vi "5-CopyFileContent.vi"() -> ()   [LabVIEW 2016, in "TestVIs.lvlib"]
uses:
  TestVIs.lvlib
panel:
  in  "Empty File":path=path "D:/Git/CSPP_MessageMaker/_CSPP_MessageMaker/TestVIs/TestTarget.vi"
  in  "File to Copy":path
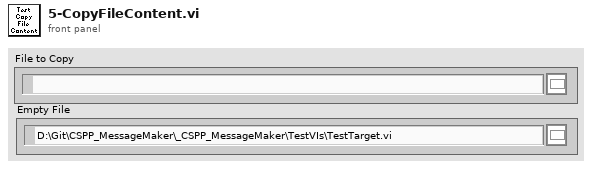
[diagram p1: front panel]
types:
  T1 = enum16{"Invalid Wire Rule", "Required", "Recommended", "Optional", "Dynamic Dispatch"}[]
  T2 = typedef "LVPositionTypeDef.ctl" = cluster{"Left":i32, "Top":i32}
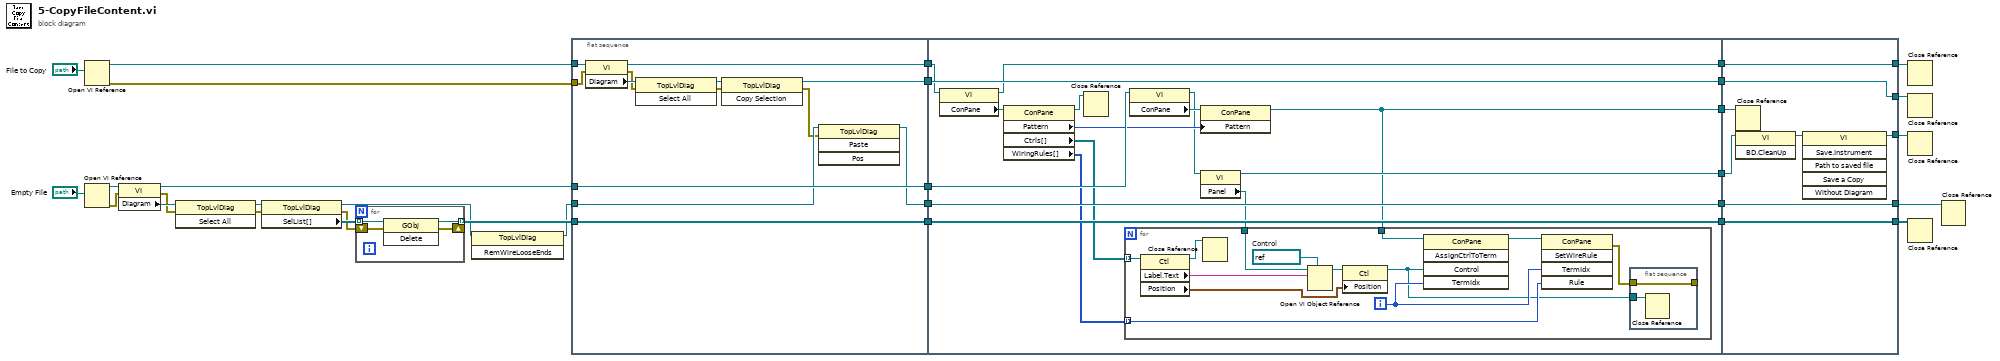
[diagram p0: block diagram]
diagram:
  n1 = Open VI Reference(vi path="File to Copy") -> (vi reference=w22:refnum<vi>, error out=w21:errorcluster)  [unwired: 5 in]
  n2 = Open VI Reference(vi path="Empty File") -> (vi reference=w31:refnum<vi>, error out=w24:errorcluster)  [unwired: 5 in]
  n3 = property class="VI"(reference=w31, error in=w24) -> (reference out=w19:refnum<vi>, error out=w29:errorcluster, "Diagram"=w30:refnum<vi>)
  n4 = invoke class="TopLvlDiag" method="Select All"(reference=w30, error in=w29) -> (reference out=w28:refnum<vi>, error out=w27:errorcluster)  [unwired: 1 in, 1 out]
  n5 = property class="TopLvlDiag"(reference=w28, error in=w27) -> (reference out=w3:refnum<vi>, error out=w25:errorcluster, "SelList[]"=w26:refnum<vi>[])
  n6 = for {
    tunnel: w26 -> [w36] mode=indexing
    shift-right: [w34] -> _
    shift-left: w25 -> [w35]
    tunnel: [w33] -> w20 mode=indexing
    n7 = invoke class="GObj" method="Delete"(reference=w36, error in=w35) -> (reference out=w33:refnum<vi>, error out=w34:errorcluster)  [unwired: 1 in, 1 out]
  }
  n8 = invoke class="TopLvlDiag" method="RemWireLooseEnds"(reference=w3) -> (reference out=w2:refnum<vi>)  [unwired: 2 in, 2 out]
  n9 = flat-sequence {
    tunnel: w22 -> [w49]
    tunnel: w21 -> [w48]
    tunnel: w2 -> [w41]
    tunnel: w20 -> [w43]
    tunnel: w19 -> [w42]
    tunnel: [w40] -> w13
    tunnel: [w43] -> w11
    tunnel: [w42] -> w9
    tunnel: [w37] -> w7
    tunnel: [w38] -> w5
    tunnel: w13 -> [w59]
    tunnel: [w59] -> w12
    tunnel: w11 -> [w65]
    tunnel: [w65] -> w10
    tunnel: w9 -> [w58]
    tunnel: [w52] -> w8
    tunnel: w7 -> [w62]
    tunnel: [w61] -> w6
    tunnel: w5 -> [w64]
    tunnel: [w64] -> w4
    tunnel: [w50] -> w1
    tunnel: [w87] -> w17
    tunnel: [w88] -> w18
    tunnel: w12 -> [w88]
    tunnel: w10 -> [w87]
    tunnel: w8 -> [w85]
    tunnel: [w84] -> w16
    tunnel: [w83] -> w15
    tunnel: w6 -> [w83]
    tunnel: [w82] -> w14
    tunnel: w4 -> [w82]
    tunnel: w1 -> [w81]
    frame #0 {
      n10 = property class="VI"(reference=w49, error in=w48) -> (reference out=w37:refnum<vi>, error out=w46:errorcluster, "Diagram"=w47:refnum<vi>)
      n11 = invoke class="TopLvlDiag" method="Select All"(reference=w47, error in=w46) -> (reference out=w45:refnum<vi>, error out=w44:errorcluster)  [unwired: 1 in, 1 out]
      n12 = invoke class="TopLvlDiag" method="Copy Selection"(reference=w45, error in=w44) -> (reference out=w38:refnum<vi>, error out=w39:errorcluster)  [unwired: 1 in, 1 out]
      n13 = invoke class="TopLvlDiag" method="Paste"(reference=w41, error in=w39) -> (reference out=w40:refnum<vi>)  [unwired: 2 in, 3 out]
    }
    frame #1 {
      n14 = property class="VI"(reference=w62) -> (reference out=w61:refnum<vi>, "ConPane"=w63:refnum<vi>)  [unwired: 1 in, 1 out]
      n15 = property class="ConPane"(reference=w63) -> (reference out=w57:refnum<vi>, "Pattern"=w56:u32, "Ctrls[]"=w55:refnum<vi>[], "WiringRules[]"=w54:T1)  [unwired: 1 in, 1 out]
      n16 = Close Reference(reference=w57) -> ()  [unwired: 1 in, 1 out]
      n17 = property class="VI"(reference=w58) -> (reference out=w53:refnum<vi>, "ConPane"=w60:refnum<vi>)  [unwired: 1 in, 1 out]
      n18 = property class="ConPane"(reference=w60, "Pattern"=w56) -> (reference out=w50:refnum<vi>)  [unwired: 1 in, 1 out]
      n19 = property class="VI"(reference=w53) -> (reference out=w52:refnum<vi>, "Panel"=w51:refnum<vi>)  [unwired: 1 in, 1 out]
      n20 = for {
        tunnel: w55 -> [w78] mode=indexing
        tunnel: w54 -> [w68] mode=indexing
        tunnel: w51 -> [w75]
        tunnel: w50 -> [w70]
        i -> [w69]
        w76 = refnum<vi> refnum  # Control
        n21 = property class="Ctl"(reference=w78) -> (reference out=w77:refnum<vi>, "Label.Text"=w74:string, "Position"=w72:T2)  [unwired: 1 in, 1 out]
        n22 = Close Reference(reference=w77) -> ()  [unwired: 1 in, 1 out]
        n23 = Open VI Object Reference(7:w76, 10:w74, 11:w75) -> (3:w73:refnum<vi>)  [unwired: 1 in, 1 out]
        n24 = property class="Ctl"(reference=w73, "Position"=w72) -> (reference out=w67:refnum<vi>)  [unwired: 1 in, 1 out]
        n25 = invoke class="ConPane" method="AssignCtrlToTerm"(reference=w70, "Control"=w67, "TermIdx"=w69) -> (reference out=w71:refnum<vi>)  [unwired: 2 in, 4 out]
        n26 = invoke class="ConPane" method="SetWireRule"(reference=w71, "TermIdx"=w69, "Rule"=w68) -> (error out=w66:errorcluster)  [unwired: 2 in, 4 out]
        n27 = flat-sequence {
          tunnel: w67 -> [w80]
          tunnel: w66 -> [w79]
          tunnel: [w79] -> _
          frame #0 {
            n28 = Close Reference(reference=w80) -> ()  [unwired: 1 in, 1 out]
          }
        }
      }
    }
    frame #2 {
      n29 = Close Reference(reference=w81) -> ()  [unwired: 1 in, 1 out]
      n30 = invoke class="VI" method="BD.CleanUp"(reference=w85) -> (reference out=w86:refnum<vi>)  [unwired: 2 in, 2 out]
      n31 = invoke class="VI" method="Save.Instrument"(reference=w86) -> (reference out=w84:refnum<vi>)  [unwired: 5 in, 5 out]
    }
  }
  n32 = Close Reference(reference=w15) -> ()  [unwired: 1 in, 1 out]
  n33 = Close Reference(reference=w14) -> ()  [unwired: 1 in, 1 out]
  n34 = Close Reference(reference=w16) -> ()  [unwired: 1 in, 1 out]
  n35 = Close Reference(reference=w17) -> ()  [unwired: 1 in, 1 out]
  n36 = Close Reference(reference=w18) -> ()  [unwired: 1 in, 1 out]
